vi "Set Marker Values.vi"(5 "Marker (1)":i32=1, 7 "Channel (1)":i32=1, 8 "error in (no error)":errorcluster, 10 "Marker To (0: Start)":u16(ring) items=["Start", "Stop", "Center", "Reference", "Electrical Delay"], 11 "VISA resource name":refnum<visa-resource-name>) -> (0 "error out":errorcluster, 3 "VISA resource name out":refnum<visa-resource-name>)   [LabVIEW 2018, in "Agilent ENA Series.lvlib"]
doc: "Sets the value of the specified item, for the active trace of selected channel, to the value of the position of selected marker."
uses:
  Agilent ENA Series.lvlib
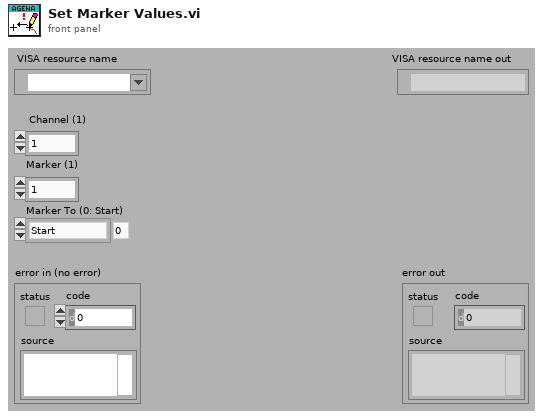
[diagram p1: front panel]
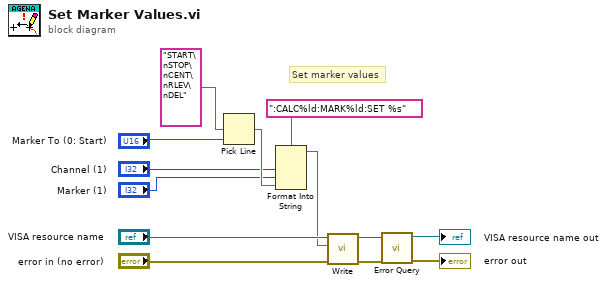
[diagram p0: block diagram]
diagram:
  # "Set marker values"
  n1 = Pick Line(multi-line string="START\nSTOP\nCENT\nRLEV\nDEL", line index="Marker To (0: Start)") -> (output string=w7:string)  [unwired: 1 in]
  n2 = Format Into String(format string=":CALC%ld:MARK%ld:SET %s", "Channel (1)", "Marker (1)", w7) -> (resulting string=w10:string)  [unwired: 2 in, 1 out]
  n3 = call "Write.vi"("error in (no error)"="error in (no error)", "String ()"=w10, "VISA resource name"="VISA resource name") -> ("error out"=w3:errorcluster, "VISA resource name out"=w4:refnum<visa-resource-name>)  [unwired: 6 in, 1 out]
  n4 = call "Error Query.vi"("error in (no error)"=w3, "VISA resource name"=w4) -> ("error out"=→"error out":errorcluster, "VISA resource name out"=→"VISA resource name out":refnum<visa-resource-name>)  [unwired: 6 in, 2 out]
